vi "Enter_Temp_Press.vi"() -> ()   [LabVIEW 2010]
uses:
  Sub VIs/ADAM Controls/Ch_description_ADAM.ctl
  Sub VIs/ADAM Controls/Module_type_ADAM.ctl
  Sub VIs/ADAM Controls/Function_ADAM.ctl
  Sub VIs/ADAM Controls/Channel_State.ctl
  Sub VIs/ADAM Controls/Calib_type_ADAM.ctl
  Sub VIs/ADAM Controls/Address.ctl
  Anemometry/Anemometry Sub Vis/File/Setup_Filetype.ctl
  Sub VIs/ADAM Controls/Channel_names.ctl
  Anemometry/Anemometry Sub Vis/Controls/Preference_Mode.ctl
  Sub VIs/ADAM Controls/Update_scan_value.ctl
  Anemometry/Anemometry Sub Vis/Globals/Preference_global.vi
  Anemometry/Anemometry Sub Vis/Globals/Constants_global.vi
panel:
  in  "OK":bool
  out "Ch Description Array":T1[](array[typedef]) {"Duty" format="%.0b"; "D" format="%#_5g"; "C" format="%#_5g"; "B" format="%#_5g"; "A" format="%#_5g"}
  in  "mbars":dbl format="%#.1f"
  in  "Deg C":dbl format="%#.1f"
  in  "type specifier VI Refnum (for type only)":refnum<vi>
  out "Preference file":path
  in  "Server Comms":T7(ring)
  in  "Browse for Atmos Press":bool
  in  "Browse for Temp Ch":bool
  in  "Flow Pressure (Absolute) (mbars)":string="Froude:NPL:Atmos_Press"
  in  "Flow Temperature (deg C)":string="EnFlo Tun:Inlet Heater:Av Temp"
  # "DATA SOURCE"
  # "CURRENT VALUES"
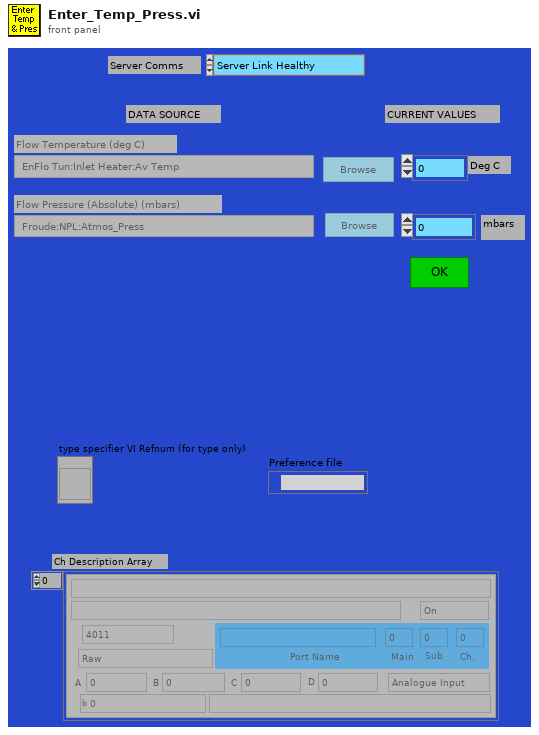
[diagram p1: front panel]
types:
  T1 = typedef "Ch_description_ADAM.ctl" = cluster{"Ch Name":string, "Type":T2, "Function":T3, "Ch State":T4, "Calibration type":T5, "A":dbl, "B":dbl, "C":dbl, "D":dbl, "Comments":string, "Address":T6, "String":string, "Duty":u16}
  T2 = typedef "Module_type_ADAM.ctl" = enum16{"4011", "4012", "4013", "4014", "4016", "4017", "4018", "4021", "4050", "4052", "4053", "4060", "4080", "5000", "5017", "5018", "5024", "5051", "5056", "5060", "6060", "Tracker", "WEST", "GILL", "JEM", "VICI", "Vaisala", "DRUCK", "Run VI Named:", "IR2100", "PPT", "Comparator", "VIRTUAL", "Hold Value", "Read A", "Read Ch", "Coded", "Client Info", "Web Client", "X10", "Test"}
  T3 = typedef "Function_ADAM.ctl" = enum16{"Analogue Input", "Digital Input", "Event counter", "Event rate", "Analogue Output", "Digital Output", "Relay Output"}
  T4 = typedef "Channel_State.ctl" = enum16{"On", "Off", "Always On", "Always Off"}
  T5 = typedef "Calib_type_ADAM.ctl" = enum16{"Raw", "Bx + A", "Cx^2 + Bx + A", "Dx^3 + Cx^2 + Bx + A", "In Band", "Hi-Tec Q", "Hi-Tec M_dot", "Text"}
  T6 = typedef "Address.ctl" = cluster{"Main":i32, "Ch.":i32, "Sub":i32, "Port Name":string}
  T7 = enum16{"Server Link Healthy", "Do Not Link To Server"}
  T8 = typedef "Setup_Filetype.ctl" = enum16{"Measurement Setups", "Calibration Setups", "General", "Results File Plotter Setups", "Speed Calib Tweaks"}
  T9 = typedef "Channel_names.ctl" = enum16{"Active Only", "Active + Off", "All Channels"}
  T10 = enum16{"Zero or one", "One", "Zero or more", "One or more"}
  T11 = typedef "Preference_Mode.ctl" = enum16{"Load Preferences from file", "Save Preferences to file", "Load, Edit then Save"}
  T12 = typedef "Server_Comms.ctl" = enum16{"Server Link Healthy", "Do Not Link To Server"}
  T13 = typedef "Update_scan_value.ctl" = cluster{"Channel Name":string, "New Value":dbl}
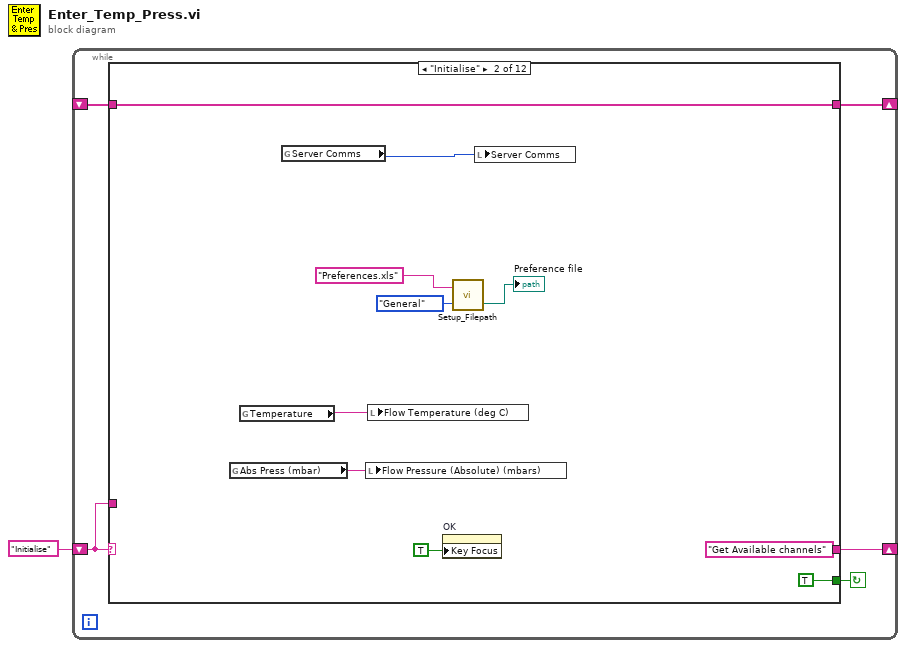
[diagram p0: block diagram]
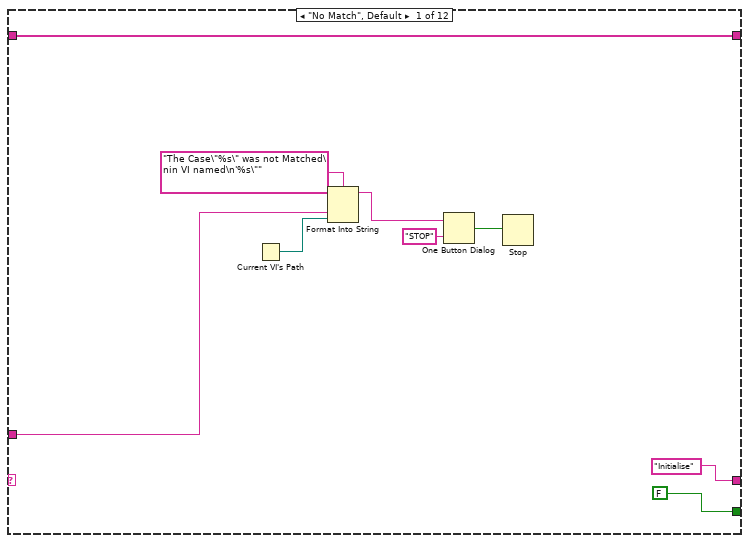
[diagram p2: hidden frame]
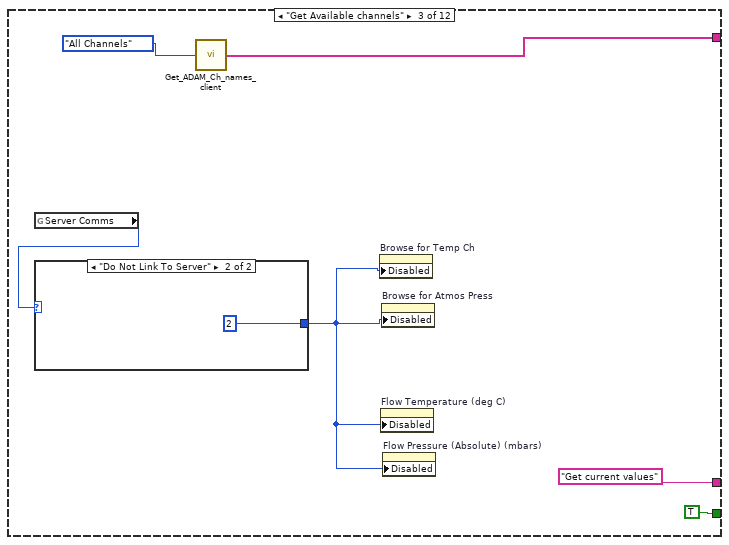
[diagram p3: hidden frame]
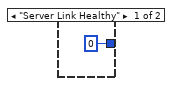
[diagram p4: hidden frame]
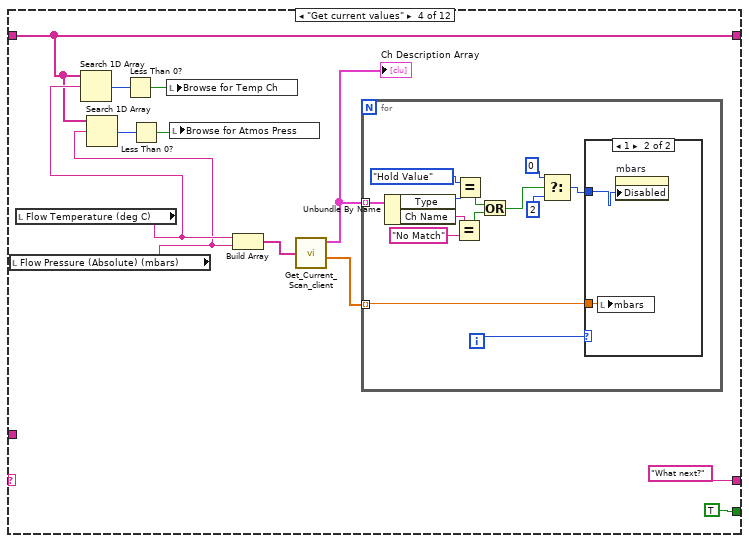
[diagram p5: hidden frame]
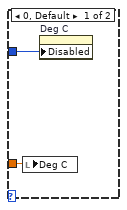
[diagram p6: hidden frame]
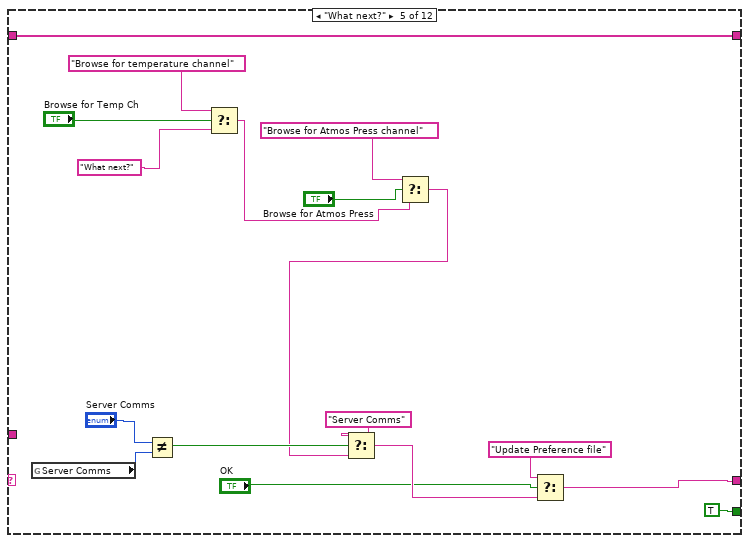
[diagram p7: hidden frame]
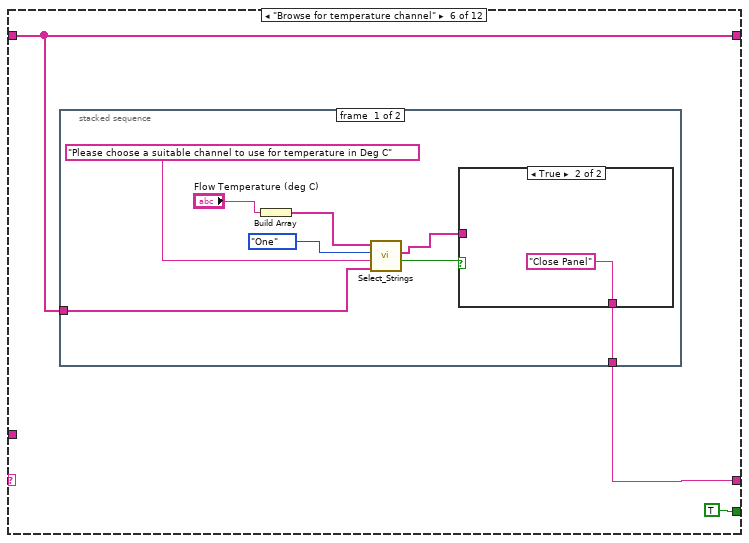
[diagram p8: hidden frame]
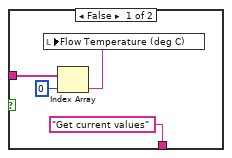
[diagram p9: hidden frame]
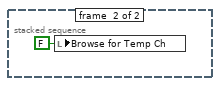
[diagram p10: hidden frame]
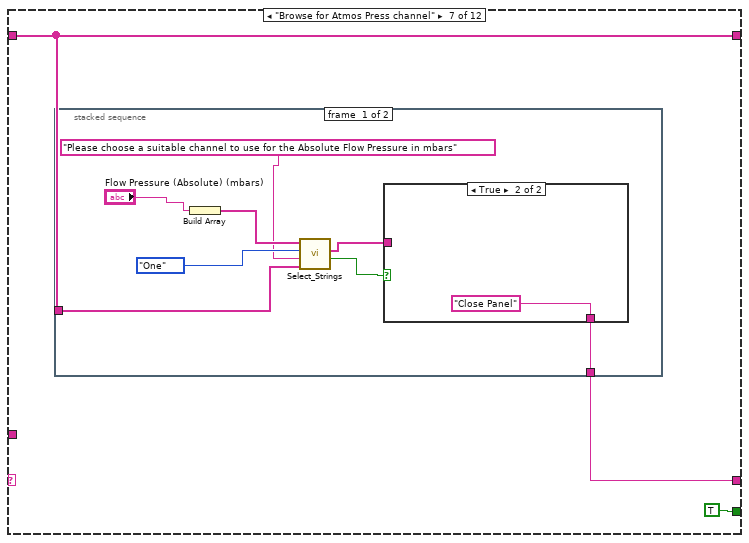
[diagram p11: hidden frame]
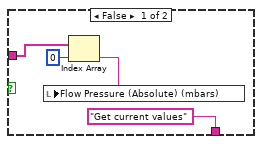
[diagram p12: hidden frame]
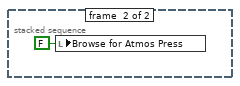
[diagram p13: hidden frame]
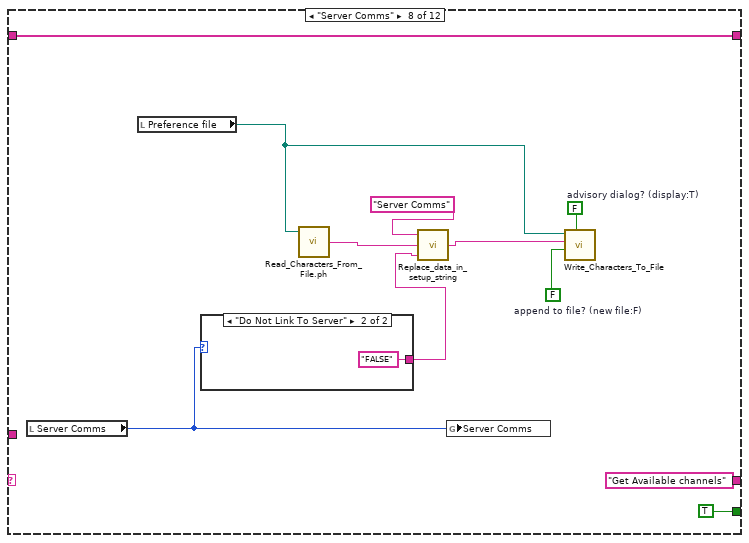
[diagram p14: hidden frame]
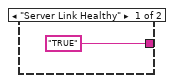
[diagram p15: hidden frame]
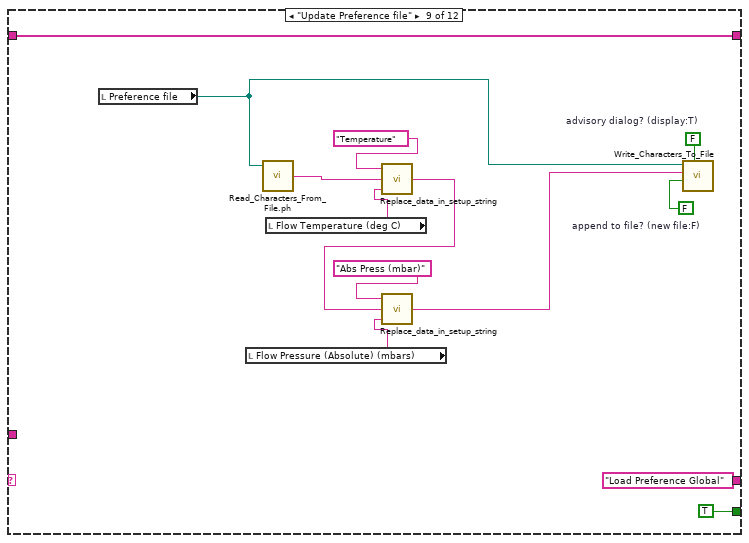
[diagram p16: hidden frame]
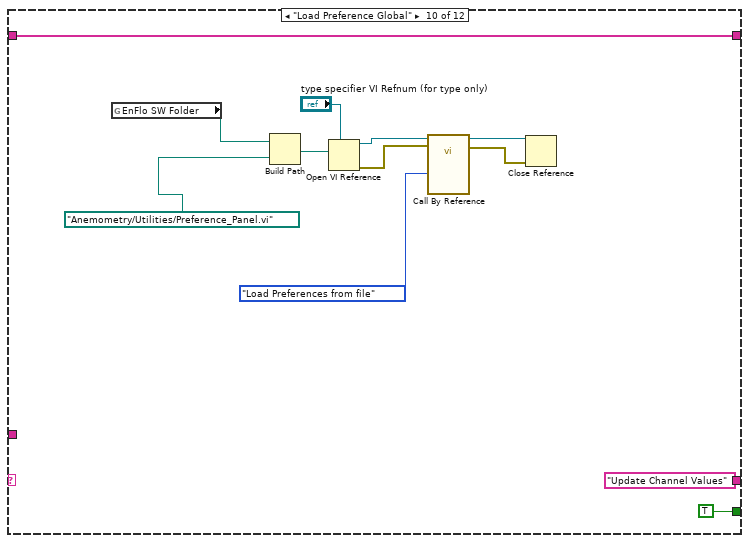
[diagram p17: hidden frame]
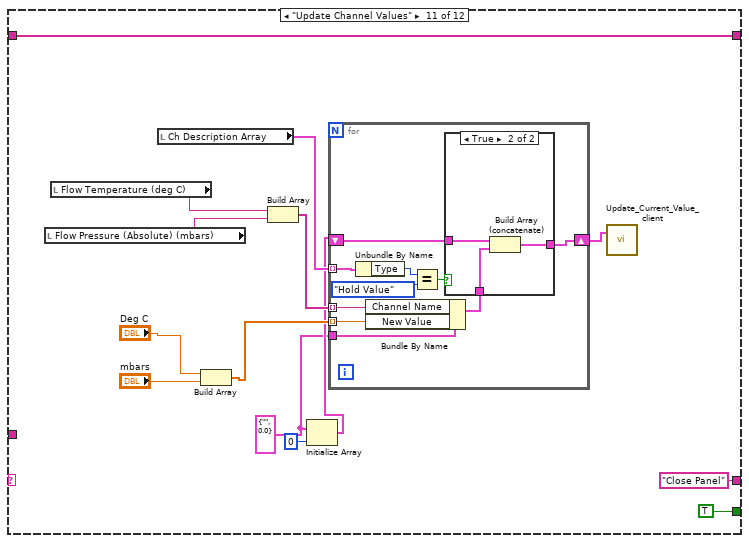
[diagram p18: hidden frame]
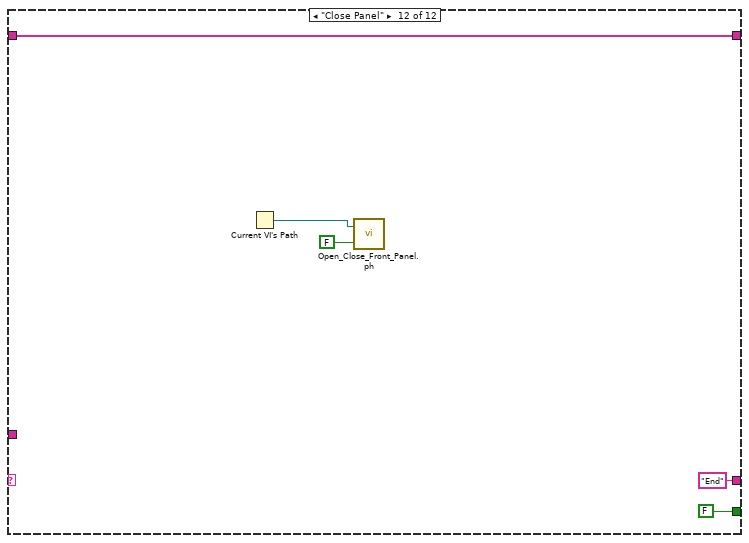
[diagram p20: hidden frame]
diagram:
  n1 = while {
    shift-left: "Initialise" -> [w4]
    shift-right: [w5] -> _
    shift-right: [w3] -> _
    shift-left: _ -> [w2]
    stop <- w6 continue-if-true
    n2 = case shown="\"Initialise\"" w4 {
      tunnel: [FALSE TRUE TRUE TRUE TRUE TRUE TRUE TRUE TRUE TRUE TRUE FALSE] -> w6
      tunnel: ["Initialise" "Get Available channels" "Get current values" "What next?" w76 w80 w97 "Get Available channels" "Load Preference Global" "Update Channel Values" "Close Panel" "End"] -> w5
      tunnel: w4 -> [w10 _ _ _ _ _ _ _ _ _ _ _]
      tunnel: [w7 w24 w28 w35 w73 w81 w98 w122 w137 w149 w163 w182] -> w3
      tunnel: w2 -> [w7 w24 _ w35 w73 w81 w98 w122 w137 w149 w163 w182]
      frame "No Match", Default {
        n3 = Current VI's Path() -> (path=w9:path)
        n4 = Format Into String(format string="The Case\"%s\" was not Matched\nin VI named\n'%s\"" ("Format String"), w10, w9) -> (resulting string=w13:string)  [unwired: 2 in, 1 out]
        n5 = One Button Dialog(message=w13, button name ("OK")="STOP") -> (true=w11:bool)
        n6 = Stop(stop? (T)=w11) -> ()
      }
      frame "Initialise" {
        n7 = global read "Preference_global.vi" "Abs Press (mbar)"() -> (w21:string)
        n8 = global read "Preference_global.vi" "Temperature"() -> (w20:string)
        n9 = global read "Preference_global.vi" "Server Comms"() -> (w25:T12)
        n10 = local write "Flow Pressure (Absolute) (mbars)"(w21) -> ()
        n11 = local write "Flow Temperature (deg C)"(w20) -> ()
        n12 = property on="OK" class="Bool"("Key Focus"=TRUE) -> ()  [unwired: 2 in, 2 out]
        n13 = call "Setup_Filepath.vi"("Setup File Type"=Setup_Filetype."General", "Filename in"="Preferences.xls" ("name or relative path")) -> ("Filename Out"=→"Preference file":path)  [unwired: 1 out]
        n14 = local write "Server Comms"(w25) -> ()
      }
      frame "Get Available channels" {
        n15 = global read "Preference_global.vi" "Server Comms"() -> (w27:T12)
        n16 = case shown="\"Do Not Link To Server\"" w27 {
          tunnel: [u8 0 ("Disabled") u8 2 ("Disabled")] -> w26
          frame "Server Link Healthy" {
          }
          frame "Do Not Link To Server" {
          }
        }
        n17 = call "Get_ADAM_Ch_names_client.vi"("Channel names set"=Channel_names."All Channels") -> ("Ch names"=w28:string[])
        n18 = property on="Browse for Temp Ch" class="Bool (strict)"("Disabled"=w26) -> ()  [unwired: 2 in, 2 out]
        n19 = property on="Flow Temperature (deg C)" class="Str"("Disabled"=w26) -> ()  [unwired: 2 in, 2 out]
        n20 = property on="Browse for Atmos Press" class="Bool (strict)"("Disabled"=w26) -> ()  [unwired: 2 in, 2 out]
        n21 = property on="Flow Pressure (Absolute) (mbars)" class="Str"("Disabled"=w26) -> ()  [unwired: 2 in, 2 out]
      }
      frame "Get current values" {
        n22 = local read "Flow Pressure (Absolute) (mbars)"() -> (w34:string)
        n23 = local read "Flow Temperature (deg C)"() -> (w40:string)
        n24 = Search 1D Array(1D array=w35, element=w40) -> (index of element=w39:i32)  [unwired: 1 out]
        n25 = Search 1D Array(1D array=w35, element=w34) -> (index of element=w38:i32)  [unwired: 1 out]
        n26 = Less Than 0?(x=w39) -> (x < 0?=w37:bool)
        n27 = Less Than 0?(x=w38) -> (x < 0?=w36:bool)
        n28 = local write "Browse for Temp Ch"(w37) -> ()
        n29 = local write "Browse for Atmos Press"(w36) -> ()
        n30 = Build Array(w40, w34) -> (w43:string[])
        n31 = call "Get_Current_Scan_client.vi"("ADAM Ch Names"=w43) -> ("Ch Description Array"=w41:T1[], "Numerical Values"=w42:dbl[])  [unwired: 1 in, 1 out]
        "Ch Description Array" <- w41
        n32 = for {
          tunnel: w42 -> [w46] mode=indexing
          tunnel: w41 -> [w57] mode=indexing
          i -> [w58]
          n33 = Unbundle By Name(w57) -> ("Type"=w56:T2, "Ch Name"=w51:string)
          n34 = Equal?(x=w51, y="No Match") -> (x = y?=w49:bool)
          n35 = Equal?(x=Module_type_ADAM."Hold Value" ("Type"), y=w56) -> (x = y?=w48:bool)
          n36 = Or(x=w48, y=w49) -> (x .or. y?=w47:bool)
          n37 = Select(t=u8 0 ("Disabled"), s=w47, f=u8 2 ("Disabled")) -> (s? t:f=w52:u8)
          n38 = case shown="1" w58 {
            tunnel: w46 -> [w60 w62]
            tunnel: w52 -> [w59 w61]
            frame 0, Default {
              n39 = local write "Deg C"(w60) -> ()
              n40 = property on="Deg C" class="DigNum (strict)"("Disabled"=w59) -> ()  [unwired: 2 in, 2 out]
            }
            frame 1 {
              n41 = local write "mbars"(w62) -> ()
              n42 = property on="mbars" class="DigNum (strict)"("Disabled"=w61) -> ()  [unwired: 2 in, 2 out]
            }
          }
        }
      }
      frame "What next?" {
        n43 = global read "Preference_global.vi" "Server Comms"() -> (w67:T12)
        n44 = Not Equal?(x="Server Comms", y=w67) -> (x != y?=w65:bool)
        n45 = Select(t="Browse for temperature channel", s="Browse for Temp Ch", f="What next?") -> (s? t:f=w70:string)
        n46 = Select(t="Browse for Atmos Press channel", s="Browse for Atmos Press", f=w70) -> (s? t:f=w63:string)
        n47 = Select(t="Server Comms", s=w65, f=w63) -> (s? t:f=w69:string)
        n48 = Select(t="Update Preference file", s="OK", f=w69) -> (s? t:f=w76:string)
      }
      frame "Browse for temperature channel" {
        n49 = stacked-sequence {
          tunnel: w81 -> [w88 _]
          tunnel: [w83 _] -> w80
          frame #0 {
            n50 = Build Array("Flow Temperature (deg C)") -> (w90:string[])
            n51 = call "Select_Strings.vi"("Available Ch names"=w88, "Message"="Please choose a suitable channel to use for temperature in Deg C", "Selector mode"=T10."One", "Desired Ch names (in)"=w90) -> ("Cancel"=w84:bool, "Selected Channel Names"=w87:string[])  [unwired: 3 out]
            n52 = case shown="True" w84 {
              tunnel: w87 -> [w94 _]
              tunnel: ["Get current values" "Close Panel"] -> w83
              frame False {
                n53 = Index Array(array=w94, index=0) -> (element=w92:string)
                n54 = local write "Flow Temperature (deg C)"(w92) -> ()
              }
              frame True {
              }
            }
          }
          frame #1 {
            n55 = local write "Browse for Temp Ch"(FALSE ("Browse for Temp Ch")) -> ()
          }
        }
      }
      frame "Browse for Atmos Press channel" {
        n56 = stacked-sequence {
          tunnel: w98 -> [w105 _]
          tunnel: [w100 _] -> w97
          frame #0 {
            n57 = Build Array("Flow Pressure (Absolute) (mbars)") -> (w107:string[])
            n58 = call "Select_Strings.vi"("Available Ch names"=w105, "Message"="Please choose a suitable channel to use for the Absolute Flow Pressure in mbars", "Selector mode"=T10."One", "Desired Ch names (in)"=w107) -> ("Cancel"=w101:bool, "Selected Channel Names"=w104:string[])  [unwired: 3 out]
            n59 = case shown="True" w101 {
              tunnel: w104 -> [w111 _]
              tunnel: ["Get current values" "Close Panel"] -> w100
              frame False {
                n60 = Index Array(array=w111, index=0) -> (element=w109:string)
                n61 = local write "Flow Pressure (Absolute) (mbars)"(w109) -> ()
              }
              frame True {
              }
            }
          }
          frame #1 {
            n62 = local write "Browse for Atmos Press"(FALSE ("Browse for Atmos Press")) -> ()
          }
        }
      }
      frame "Server Comms" {
        w121 = FALSE  # append to file? (new file:F)
        w120 = FALSE  # advisory dialog? (display:T)
        n63 = local read "Server Comms"() -> (w115:T7)
        n64 = local read "Preference file"() -> (w117:path)
        n65 = case shown="\"Do Not Link To Server\"" w115 {
          tunnel: ["TRUE" "FALSE"] -> w114
          frame "Server Link Healthy" {
          }
          frame "Do Not Link To Server" {
          }
        }
        n66 = call "Read_Characters_From_File.ph.vi"("file path (dialog if empty)"=w117) -> ("character string"=w119:string)  [unwired: 1 in, 7 out]
        n67 = call "Replace_data_in_setup_string.vi"("New data string"=w114, "Input string"=w119, "Variable name"="Server Comms") -> ("Appended string"=w118:string)
        n68 = global write "Preference_global.vi" "Server Comms"(w115) -> ()
        n69 = call "Write_Characters_To_File.vi"("file path (dialog if empty)"=w117, "advisory dialog? (display:T)"=w120, "character string"=w118, "append to file? (new file:F)"=w121) -> ()  [unwired: 1 in, 4 out]
      }
      frame "Update Preference file" {
        w136 = FALSE  # append to file? (new file:F)
        w135 = FALSE  # advisory dialog? (display:T)
        n70 = local read "Preference file"() -> (w133:path)
        n71 = local read "Flow Pressure (Absolute) (mbars)"() -> (w130:string)
        n72 = call "Read_Characters_From_File.ph.vi"("file path (dialog if empty)"=w133) -> ("character string"=w134:string)  [unwired: 1 in, 7 out]
        n73 = local read "Flow Temperature (deg C)"() -> (w131:string)
        n74 = call "Replace_data_in_setup_string.vi"("New data string"=w131, "Input string"=w134, "Variable name"="Temperature") -> ("Appended string"=w128:string)
        n75 = call "Replace_data_in_setup_string.vi"("New data string"=w130, "Input string"=w128, "Variable name"="Abs Press (mbar)") -> ("Appended string"=w127:string)
        n76 = call "Write_Characters_To_File.vi"("file path (dialog if empty)"=w133, "advisory dialog? (display:T)"=w135, "character string"=w127, "append to file? (new file:F)"=w136) -> ()  [unwired: 1 in, 4 out]
      }
      frame "Load Preference Global" {
        n77 = global read "Constants_global.vi" "EnFlo SW Folder"() -> (w142:path)
        n78 = Build Path(base path=w142, name or relative path=path "Anemometry/Utilities/Preference_Panel.vi") -> (appended path=w144:path)
        n79 = Open VI Reference(type specifier VI Refnum (for type only)="type specifier VI Refnum (for type only)", vi path=w144) -> (vi reference=w145:refnum<vi>, error out=w146:errorcluster)  [unwired: 1 in, 3 out]
        n80 = call-by-ref "?"(reference=w145, error in=w146, "Mode"=Preference_Mode."Load Preferences from file") -> (reference out=w147:refnum<vi>, error out=w148:errorcluster)
        n81 = Close Reference(reference=w147, error in (no error)=w148) -> ()  [unwired: 1 out]
      }
      frame "Update Channel Values" {
        w153 = T13 {"Channel Name"="", "New Value"=0.0} ("Update Scan Value Cluster")
        n82 = local read "Flow Pressure (Absolute) (mbars)"() -> (w160:string)
        n83 = local read "Flow Temperature (deg C)"() -> (w159:string)
        n84 = local read "Ch Description Array"() -> (w156:T1[])
        n85 = Build Array("Deg C", "mbars") -> (w157:dbl[])
        n86 = Build Array(w159, w160) -> (w158:string[])
        n87 = Initialize Array(w153, 0 ("dimension size")) -> (w154:T13[])
        n88 = for {
          shift-right: [w167] -> w152
          shift-left: w154 -> [w169]
          tunnel: w158 -> [w175] mode=indexing
          tunnel: w157 -> [w174] mode=indexing
          tunnel: w156 -> [w173] mode=indexing
          tunnel: w153 -> [w166]
          n89 = Unbundle By Name(w173) -> ("Type"=w171:T2)
          n90 = Bundle By Name(cluster=w166, "Channel Name"=w175, "New Value"=w174) -> (w168:T13)
          n91 = Equal?(x=w171, y=Module_type_ADAM."Hold Value" ("Type")) -> (x = y?=w170:bool)
          n92 = case shown="True" w170 {
            tunnel: w169 -> [w176 w179]
            tunnel: w168 -> [_ w178]
            tunnel: [w176 w177] -> w167
            frame False {
            }
            frame True {
              n93 = Build Array (concatenate)(w179, w178) -> (w177:T13[])
            }
          }
        }
        n94 = call "Update_Current_Value_client.vi"("Update array in"=w152) -> ()  [unwired: 1 in]
      }
      frame "Close Panel" {
        n95 = Current VI's Path() -> (path=w181:path)
        n96 = call "Open_Close_Front_Panel.ph.vi"("Front Panel Window:Open"=FALSE, "VI path"=w181) -> ()  [unwired: 2 out]
      }
    }
  }
